vi "Destroy.vi"(8 "error in (no error)":errorcluster, 11 "NetworkConnection in":refnum<class "NetworkConnection.lvclass">) -> (0 "error out":errorcluster, 3 "NetworkConnection out":refnum<class "NetworkConnection.lvclass">)   [LabVIEW 2020, in "NetworkConnection.lvclass"]
doc: "Performs the required cleanup for the instance of the Network Connection.\n\nJKI Network Streams Connection 1.1.1.15\nJavier Ruiz - JKI\nCopyright (c) 2020, JKI\n\nThis library is provided \"AS IS\" ,WITHOUT WARRANTIES OR CONDITIONS OF ANY KIND, either express or implied."
uses:
  NetworkConnection.lvclass
  NetworkMessage--Cluster.ctl
  NetworkCommand--Cluster.ctl
  NetworkConnection.lvclass/NetworkConnection.ctl
panel:
  # "Copyright © 2020 JKI All rights reserved.\n\nAuthor: Javier Ruiz <javier.ruiz@jki.net>\n\nThis library is provided \"AS IS\" ,WITHOUT WARRANTIES OR \nCONDITIONS OF ANY KIND, either expressed or implied.\n\nJKI -- jki.net"
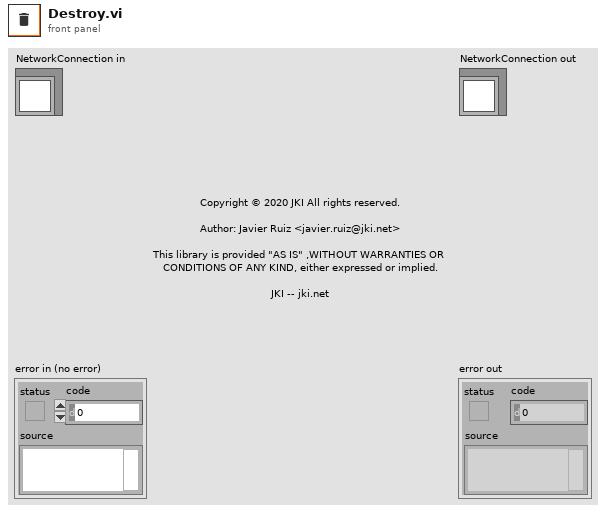
[diagram p1: front panel]
types:
  T1 = typedef "NetworkConnection.lvclass/NetworkMessage--Cluster.ctl" = cluster{"NetworkCommand":T2, "Wait for Ack?":bool, "Ack Id":i32}
  T2 = typedef "NetworkConnection.lvclass/NetworkCommand--Cluster.ctl" = cluster{"Command":string, "Arguments":variant, " Msg Id":i32}
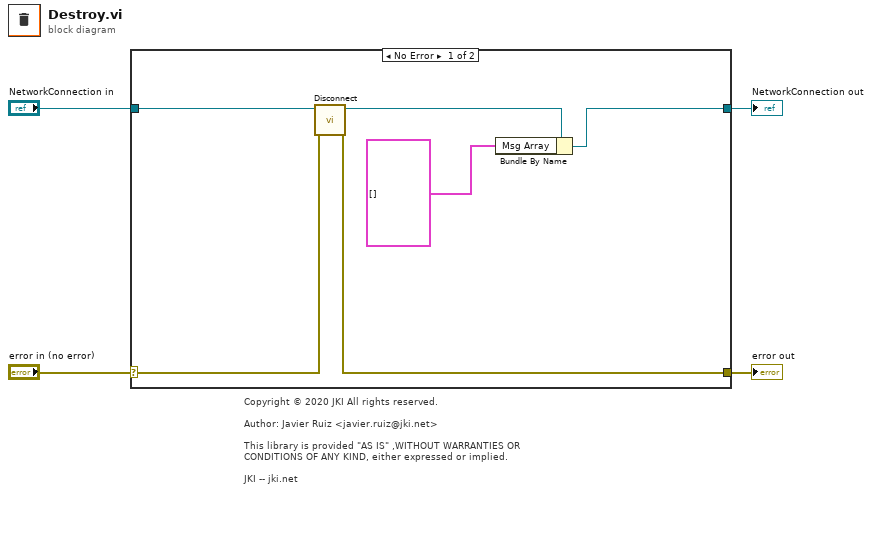
[diagram p0: block diagram]
diagram:
  # "Copyright © 2020 JKI All rights reserved.\n\nAuthor: Javier Ruiz <javier.ruiz@jki.net>\n\nThis library is provided \"AS IS\" ,WITHOUT WARRANTIES OR \nCONDITIONS OF ANY KIND, either expressed or implied.\n\nJKI -- jki.net"
  n1 = case shown="No Error" "error in (no error)" {
    selector: "error in (no error)" -> [w9 w12]
    tunnel: [w8 w12] -> w3
    tunnel: [w6 w11] -> w1
    tunnel: "NetworkConnection in" -> [w10 w11]
    frame No Error {
      n2 = call "Disconnect.vi"("error in (no error)"=w9, "NetworkConnection in"=w10) -> ("error out"=w8:errorcluster, "NetworkConnection out"=w7:refnum<class "NetworkConnection.lvclass">)  [unwired: 8 in]
      n3 = Bundle By Name(cluster=w7, "Msg Array"=T1[] []) -> (w6:refnum<class "NetworkConnection.lvclass">)
    }
    frame Error {
    }
  }
  "error out" <- w3
  "NetworkConnection out" <- w1
